vi "Calc Delays.vi"(9 "Max Delay (µs)":dbl=0.067, 10 "AB Width (ns)":dbl=19.0 min=4.0 format="%.4f", 11 "AB Delay (ns)":dbl=13.0 min=0.0 max=100000000.0 format="%.4f") -> (0 "B Delay (µs)":dbl format="%.4f", 1 "A Output Offset":u32, 2 "A Width µs)":dbl format="%.4f", 3 "A Delay 1 (µs)":dbl format="%.4f", 4 "B Output Offset":u32, 5 "Longest Delay (ns)":dbl)   [LabVIEW 2009]
panel:
  # "NOTICE -- YOU MUST LEAVE THIS NOTICE IN PLACE.  PER THE TERMS OF THE LICENSE BELOW, YOU MAY SUBLICENSE THIS SOFTWARE \nIN ANY WAY THAT DOES NOT CONFLICT WITH THIS LICENSE.\n\n### BSD License (http://www.opensource.org/licenses/bsd-license.php) Begin ###\n \nCopyright (c) 2011, Applied Energetics, http://www.appliedenergetics.com,\n                               Richard Schwerdtfeger, <rschwerdtfeger@appliedenergetics.com>\n\nAll rights reserved.\n\nRedistribution and use in source and binary forms, with or without modification, are permitted provided that the \nfollowing conditions are met:\n\n    * Redistributions of source code must retain the above copyright notice, this list of conditions and the following disclaimer.\n    * Redistributions in binary form must reproduce the above copyright notice, this list of conditions and the following disclaimer \n       in the documentation and/or other materials provided with the distribution.\n    * Neither the name of Richard Schwerdtfeger, Applied Energetics, Inc., nor the names of its contributors may be used to \n       endorse or promote products derived from this software without specific prior written permission.\n\nTHIS SOFTWARE IS PROVIDED BY THE COPYRIGHT HOLDERS AND CONTRIBUTORS \"AS IS\" AND ANY EXPRESS OR IMPLIED WARRANTIES, \nINCLUDING, BUT NOT LIMITED TO, THE IMPLIED WARRANTIES OF MERCHANTABILITY AND FITNESS FOR A PARTICULAR PURPOSE ARE \nDISCLAIMED. IN NO EVENT SHALL THE COPYRIGHT OWNER OR CONTRIBUTORS BE LIABLE FOR ANY DIRECT, INDIRECT, INCIDENTAL,\n SPECIAL, EXEMPLARY, OR CONSEQUENTIAL DAMAGES (INCLUDING, BUT NOT LIMITED TO, PROCUREMENT OF SUBSTITUTE GOODS OR \nSERVICES; LOSS OF USE, DATA, OR PROFITS; OR BUSINESS INTERRUPTION) HOWEVER CAUSED AND ON ANY THEORY OF LIABILITY, \nWHETHER IN CONTRACT, STRICT LIABILITY, OR TORT (INCLUDING NEGLIGENCE OR OTHERWISE) ARISING IN ANY WAY OUT OF THE USE \nOF THIS SOFTWARE, EVEN IF ADVISED OF THE POSSIBILITY OF SUCH DAMAGE.\n\n### BSD License End ###"
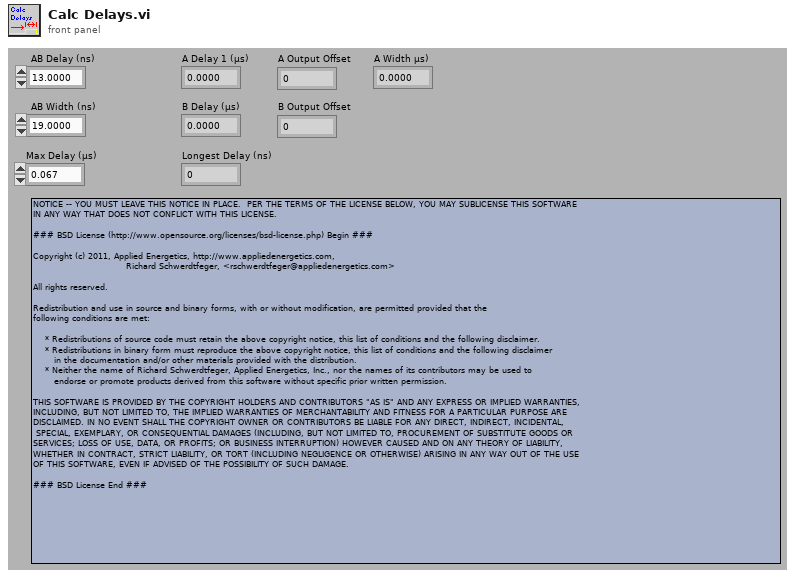
[diagram p1: front panel]
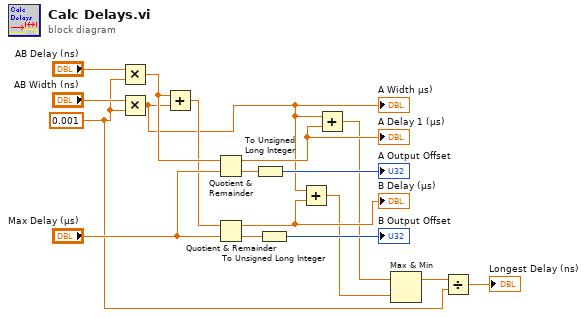
[diagram p0: block diagram]
diagram:
  w2 = 0.001 ("y")
  n1 = Multiply(x="AB Delay (ns)", y=w2) -> (x*y=w16:dbl)
  n2 = Multiply(x="AB Width (ns)", y=w2) -> (x*y=w7:dbl)
  "A Width µs)" <- w7
  n3 = Add(x=w16, y=w7) -> (x+y=w10:dbl)
  n4 = Quotient & Remainder(x=w16, y="Max Delay (µs)") -> (x-y*floor(x/y)=w8:dbl, floor(x/y)=w15:dbl)
  "A Delay 1 (µs)" <- w8
  n5 = Quotient & Remainder(x=w10, y="Max Delay (µs)") -> (x-y*floor(x/y)=w6:dbl, floor(x/y)=w13:dbl)
  "B Delay (µs)" <- w6
  n6 = To Unsigned Long Integer(number=w15) -> (unsigned 32bit integer=→"A Output Offset":u32)
  n7 = To Unsigned Long Integer(number=w13) -> (unsigned 32bit integer=→"B Output Offset":u32)
  n8 = Add(x=w7, y=w6) -> (x+y=w5:dbl)
  n9 = Add(x=w7, y=w8) -> (x+y=w4:dbl)
  n10 = Max & Min(x=w4, y=w5) -> (max(x,y)=w3:dbl)  [unwired: 1 out]
  n11 = Divide(x=w3, y=w2) -> (x/y=→"Longest Delay (ns)":dbl)
